vi "cal_main_format_node_pos.vi"(0 "Last Function Ref In":refnum<vi>, 7 "1st sub node x position":i32, 9 "Last sub node y position":i32) -> (4 "Last Function Ref Out":refnum<vi>, 6 "Main Node Position":cluster{u32, i32})   [LabVIEW 2018]
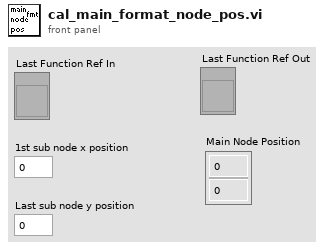
[diagram p1: front panel]
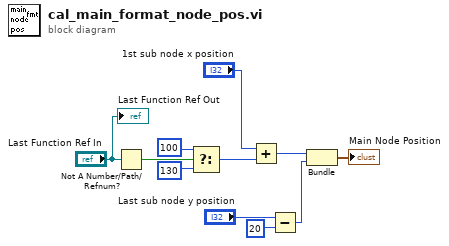
[diagram p0: block diagram]
diagram:
  n1 = Not A Number/Path/Refnum?(number/path/refnum="Last Function Ref In") -> (NaN/Path/Refnum?=w3:bool)
  n2 = Select(t=100, s=w3, f=u32 130 ("y")) -> (s? t:f=w7:u32)
  n3 = Add(x="1st sub node x position", y=w7) -> (x+y=w5:u32)
  n4 = Subtract(x="Last sub node y position", y=20) -> (x-y=w10:i32)
  n5 = Bundle(w5, w10) -> (→"Main Node Position":cluster{u32, i32})  [unwired: 1 out]
  "Last Function Ref Out" <- "Last Function Ref In"
